vi "CaptureZSpan.vi"(8 "error in (no error)":errorcluster, 9 "Center Frequency (Hz)":dbl, 10 "Sweep Time (s)":dbl, 11 "SpecA_MXA in":refnum<class "SpecA_MXA.lvclass">) -> (0 "error out":errorcluster, 2 "Captured Waveform":waveform(dbl)(graph), 3 "SpecA_MXA out":refnum<class "SpecA_MXA.lvclass">)   [LabVIEW 2014, in "SpecA_MXA.lvclass"]
uses:
  SpecA_MXA.lvclass
  SpecA_MXA.lvclass/SpecA_MXA.ctl
  <instrlib>/Agilent MXA Series/Public/Configure/Configure Frequency (Center Span).vi
  <instrlib>/Agilent MXA Series/Agilent MXA Series.lvlib
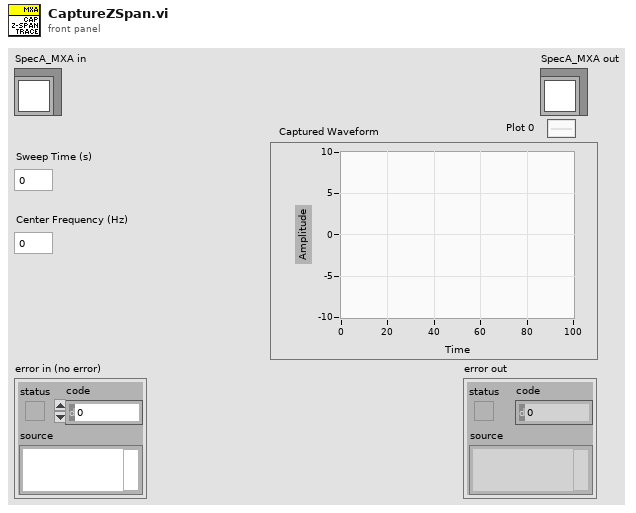
[diagram p1: front panel]
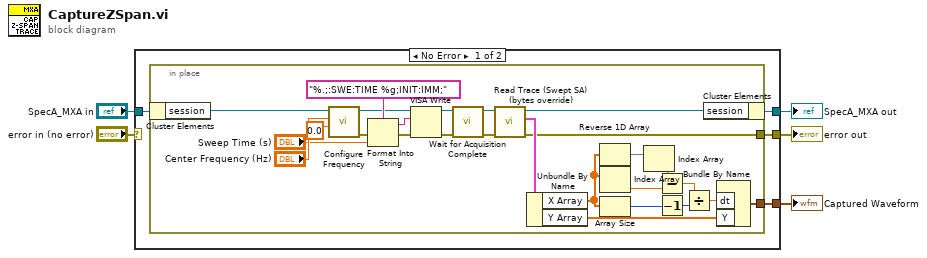
[diagram p0: block diagram]
diagram:
  n1 = case shown="No Error" "error in (no error)" {
    selector: "error in (no error)" -> [_ w37]
    tunnel: [w9 _] -> w5
    tunnel: "SpecA_MXA in" -> [w8 w36]
    tunnel: [w7 w36] -> w3
    tunnel: [w6 w37] -> w2
    frame No Error {
      n2 = in-place {
        in-place-border: [w17] -> w9
        in-place-border: [w14] -> w6
        n3 = in-place-cluster #1(w8) -> ("session"=w15:refnum<visa-resource-name>)
        n4 = call-poly <instrlib>:"Configure Frequency.vi"("Span (2.65E+10 Hz)"=0.0, "Center Frequency (1.325E+10 Hz)"="Center Frequency (Hz)", "VISA resource name"=w15) -> ("error out"=w30:errorcluster, "VISA resource name out"=w34:refnum<visa-resource-name>)  [unwired: 7 in]
        n5 = Format Into String(format string="%.;:SWE:TIME %g;INIT:IMM;", error in=w30, "Sweep Time (s)") -> (resulting string=w13:string, error out=w29:errorcluster)  [unwired: 1 in]
        n6 = VISA Write(VISA resource name=w34, write buffer=w13, error in (no error)=w29) -> (VISA resource name out=w31:refnum<visa-resource-name>, error out=w28:errorcluster)  [unwired: 1 out]
        n7 = call <instrlib>:"Wait for Acquisition Complete.vi"("error in (no error)"=w28, "VISA resource name"=w31) -> ("error out"=w33:errorcluster, "VISA resource name out"=w32:refnum<visa-resource-name>)  [unwired: 8 in]
        n8 = call "Read Trace (Swept SA) (bytes override).vi"("error in (no error)"=w33, "VISA resource name"=w32) -> ("error out"=w14:errorcluster, "Trace Waveform"=w27:cluster{"X Array":dbl[], "Y Array":dbl[]}, "VISA resource name out"=w10:refnum<visa-resource-name>)  [unwired: 7 in]
        n9 = Unbundle By Name(w27) -> ("X Array"=w21:dbl[], "Y Array"=w26:dbl[])
        n10 = Reverse 1D Array(array=w21) -> (reversed array=w25:dbl[])
        n11 = Index Array(array=w21) -> (element=w23:dbl)  [unwired: 1 in]
        n12 = Array Size(array=w21) -> (size(s)=w20:i32)
        n13 = Index Array(array=w25) -> (element=w24:dbl)  [unwired: 1 in]
        n14 = Subtract(x=w24, y=w23) -> (x-y=w22:dbl)
        n15 = Decrement(x=w20) -> (x-1=w19:i32)
        n16 = Divide(x=w22, y=w19) -> (x/y=w18:dbl)
        n17 = in-place-cluster #1("session"=w10) -> (w7:refnum<class "SpecA_MXA.lvclass">)
        n18 = Bundle By Name("dt"=w18, "Y"=w26) -> (w17:waveform(dbl))  [unwired: 1 in]
      }
    }
    frame Error {
    }
  }
  "Captured Waveform" <- w5
  "SpecA_MXA out" <- w3
  "error out" <- w2
